vi "Read SALT location.vi"(8 "error in (no error)":errorcluster, 11 "Encryption in":refnum<class "Encryption.lvclass">) -> (0 "error out":errorcluster, 2 "SALT location":u16(ring)=1 items=["both", "start of string", "end of string"], 3 "Encryption out":refnum<class "Encryption.lvclass">)   [LabVIEW 2019, in "TSC Event Logger.lvlib" / "Encryption.lvclass"]
uses:
  Encryption.lvclass
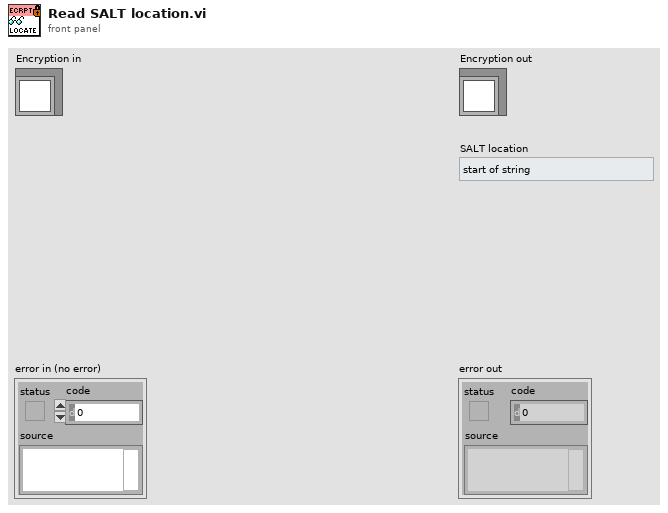
[diagram p1: front panel]
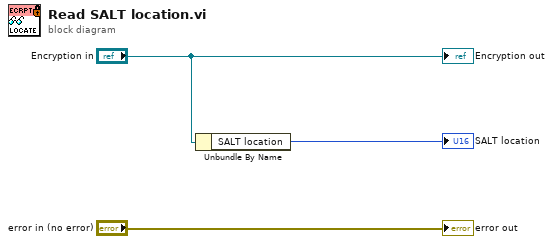
[diagram p0: block diagram]
diagram:
  n1 = Unbundle By Name("Encryption in") -> ("SALT location"=→"SALT location":u16)
  "error out" <- "error in (no error)"
  "Encryption out" <- "Encryption in"
